vi "Get CD Storage Library Loaded.vi"(11 "DMA Channel Testing in":refnum<class "FPGA Addon DMA Channel Unit Tests.lvclass">) -> (2 "CDS Loaded":bool, 3 "DMA Channel Testing out":refnum<class "FPGA Addon DMA Channel Unit Tests.lvclass">)   [LabVIEW 2018, in "FPGA Addon DMA Channel Unit Tests.lvclass"]
uses:
  FPGA Addon DMA Channel Unit Tests.lvclass
  FPGA Addon DMA Channel Unit Tests.lvclass/FPGA Addon DMA Channel Unit Tests.ctl
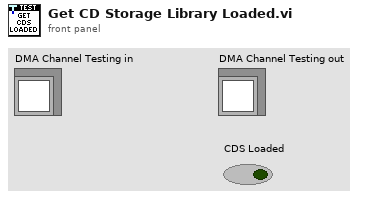
[diagram p1: front panel]
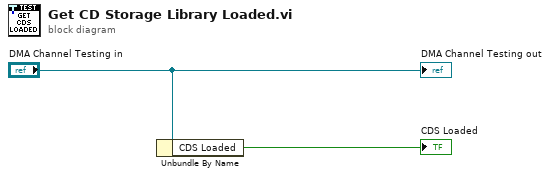
[diagram p0: block diagram]
diagram:
  n1 = Unbundle By Name("DMA Channel Testing in") -> ("CDS Loaded"=→"CDS Loaded":bool)
  "DMA Channel Testing out" <- "DMA Channel Testing in"
